vi "Means.vi"(9 "type":T1(ring), 10 "x array":dbl[](array[numeric])) -> (0 "mean value":dbl, 2 "error":i32)   [LabVIEW 2017]
uses:
  <vilib>/gmath/NI_Gmath.lvlib
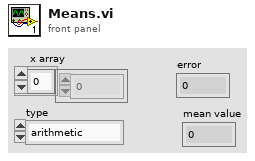
[diagram p1: front panel]
types:
  T1 = enum16{"arithmetic", "geometric", "harmonic", "trimmed", "median"}
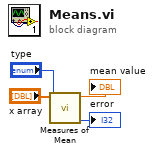
[diagram p0: block diagram]
diagram:
  n1 = call <vilib>:"Measures of Mean.vi"("type"="type", "x array"="x array") -> ("error"=→"error":i32, "mean value"=→"mean value":dbl)  [unwired: 8 in]
